vi "Method.vi"(4 "Input B":refnum<class "Abs_Numeric.lvclass">, 5 "Input A":T1) -> (1 "Result":T1)   [LabVIEW 2021, in "Divide_SGL.lvclass"]
uses:
  Divide_SGL.lvclass
  Abs Type.ctl
  Abs_Types/Single Float/Abs_Single Float.lvclass
  Abs_Types/Numeric/Abs_Numeric.lvclass
  C:/TSA/LV_Abstract/Source/Functions/Support/Function/Two Terminal/SGL/AbsFunc_Two Term_SGL.lvclass
  C:/Program Files (x86)/National Instruments/LabVIEW 2021/vi.lib/TSA/Abstract Data Classes/Abs_Types/Single Float/Abs_Single Float.lvclass
  Support/Function/Two Terminal/SGL/AbsFunc_Two Term_SGL.lvclass/AbsFunc_Two Term_SGL.ctl
  Support/Function/Two Terminal/SGL/Properties/Write Numeric A.vi
  Support/Function/Two Terminal/SGL/Properties/Write Numeric B.vi
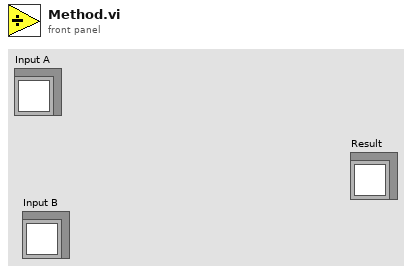
[diagram p1: front panel]
types:
  T1 = typedef "Divide_SGL.lvclass/Abs Type.ctl" = refnum<class "Abs_Single Float.lvclass">
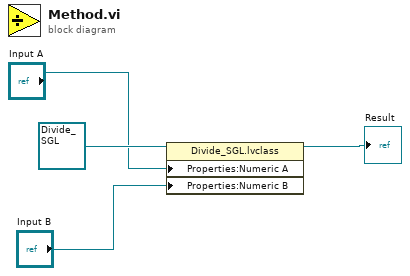
[diagram p0: block diagram]
diagram:
  n1 = property class="Divide_SGL.lvclass"(reference=refnum<class "Divide_SGL.lvclass"> refnum ("Functions.lvlib:Numeric.lvlib:Divide.lvclass"), "Properties:Numeric A"="Input A", "Properties:Numeric B"="Input B") -> (reference out=→"Result":refnum<class "Divide_SGL.lvclass">)  [unwired: 1 in, 1 out]
